vi "pelletpercents.vi"(6 "Run/Stop":bool, 8 "grading threshoulds":dbl[](array[numeric]), 11 "Sorted data":dbl[](array[numeric])) -> (2 "Percentage":dbl[](array[numeric]))   [LabVIEW 2019]
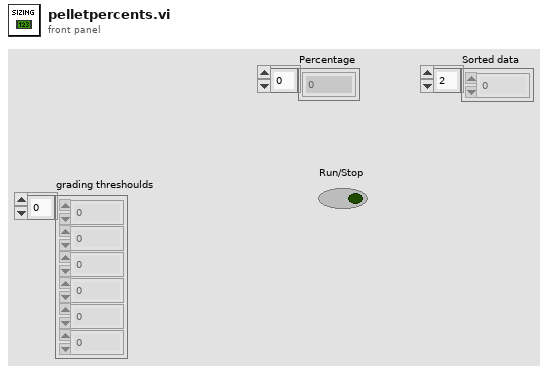
[diagram p1: front panel]
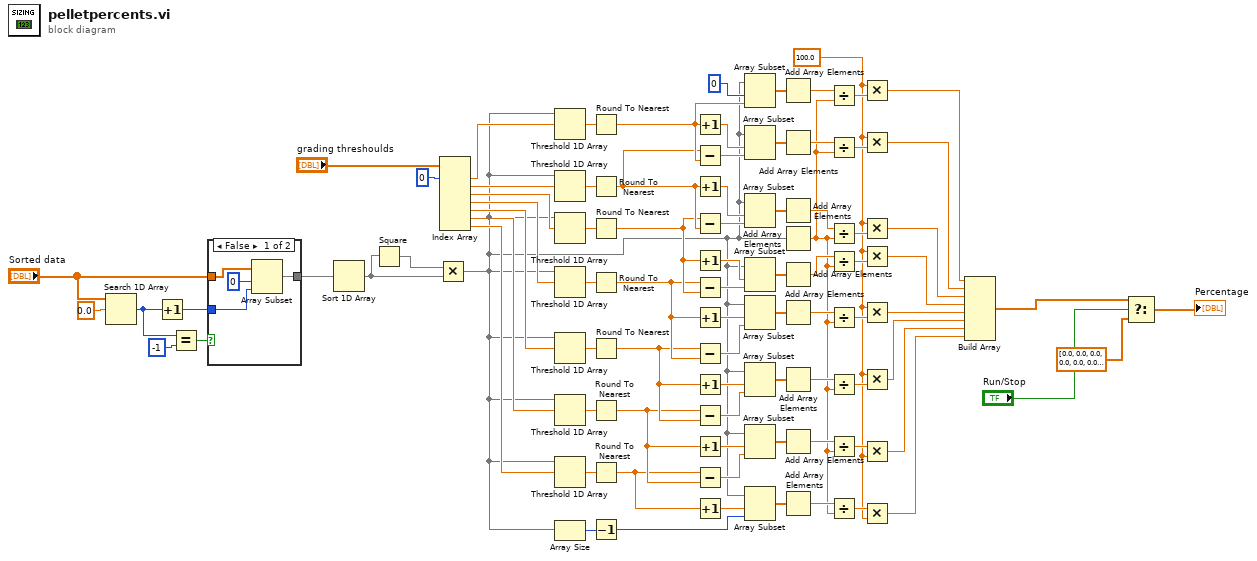
[diagram p0: block diagram]
diagram:
  w6 = 100.0 ("x")
  n1 = Search 1D Array(1D array="Sorted data", element=0.0) -> (index of element=w24:i32)  [unwired: 1 in]
  n2 = Increment(x=w24) -> (x+1=w23:i32)
  n3 = Equal?(x=w24, y=-1) -> (x = y?=w27:bool)
  n4 = case shown="False" w27 {
    tunnel: "Sorted data" -> [w91 w92]
    tunnel: [w88 w92] -> w25
    tunnel: w23 -> [w89 _]
    frame False {
      n5 = Array Subset(array=w91, index=0, length=w89) -> (w88:dbl[])
    }
    frame True {
    }
  }
  n6 = Sort 1D Array(array=w25) -> (sorted array=w30:dbl[])
  n7 = Square(x=w30) -> (x^2=w31:dbl[])
  n8 = Multiply(x=w31, y=w30) -> (x*y=w14:dbl[])
  n9 = Index Array(array="grading threshoulds", index #1=0 ("index")) -> (element #1=w22:dbl, element #2=w21:dbl, element #3=w20:dbl, element #4=w19:dbl, element #5=w18:dbl, element #6=w17:dbl, element #7=w15:dbl)  [unwired: 6 in]
  n10 = Threshold 1D Array(2:w22, 3:w14) -> (0:w79:dbl)  [unwired: 1 in]
  n11 = Threshold 1D Array(2:w21, 3:w14) -> (0:w86:dbl)  [unwired: 1 in]
  n12 = Threshold 1D Array(2:w20, 3:w14) -> (0:w85:dbl)  [unwired: 1 in]
  n13 = Threshold 1D Array(2:w19, 3:w14) -> (0:w84:dbl)  [unwired: 1 in]
  n14 = Threshold 1D Array(2:w18, 3:w14) -> (0:w83:dbl)  [unwired: 1 in]
  n15 = Threshold 1D Array(2:w17, 3:w14) -> (0:w82:dbl)  [unwired: 1 in]
  n16 = Threshold 1D Array(2:w15, 3:w14) -> (0:w16:dbl)  [unwired: 1 in]
  n17 = Array Size(array=w14) -> (size(s)=w55:i32)
  n18 = Round To Nearest(number=w79) -> (nearest integer value=w74:dbl)
  n19 = Round To Nearest(number=w86) -> (nearest integer value=w53:dbl)
  n20 = Round To Nearest(number=w85) -> (nearest integer value=w51:dbl)
  n21 = Round To Nearest(number=w84) -> (nearest integer value=w49:dbl)
  n22 = Round To Nearest(number=w83) -> (nearest integer value=w47:dbl)
  n23 = Round To Nearest(number=w82) -> (nearest integer value=w40:dbl)
  n24 = Round To Nearest(number=w16) -> (nearest integer value=w13:dbl)
  n25 = Decrement(x=w55) -> (x-1=w11:i32)
  n26 = Increment(x=w74) -> (x+1=w80:dbl)
  n27 = Subtract(x=w53, y=w74) -> (x-y=w54:dbl)
  n28 = Increment(x=w53) -> (x+1=w78:dbl)
  n29 = Subtract(x=w51, y=w53) -> (x-y=w52:dbl)
  n30 = Increment(x=w51) -> (x+1=w77:dbl)
  n31 = Subtract(x=w49, y=w51) -> (x-y=w50:dbl)
  n32 = Increment(x=w49) -> (x+1=w76:dbl)
  n33 = Subtract(x=w47, y=w49) -> (x-y=w48:dbl)
  n34 = Increment(x=w47) -> (x+1=w75:dbl)
  n35 = Subtract(x=w40, y=w47) -> (x-y=w46:dbl)
  n36 = Increment(x=w40) -> (x+1=w45:dbl)
  n37 = Subtract(x=w13, y=w40) -> (x-y=w44:dbl)
  n38 = Increment(x=w13) -> (x+1=w12:dbl)
  n39 = Array Subset(array=w14, index=0, length=w74) -> (w73:dbl[])
  n40 = Array Subset(array=w14, index=w80, length=w54) -> (w72:dbl[])
  n41 = Array Subset(array=w14, index=w78, length=w52) -> (w71:dbl[])
  n42 = Array Subset(array=w14, index=w77, length=w50) -> (w70:dbl[])
  n43 = Array Subset(array=w14, index=w76, length=w48) -> (w69:dbl[])
  n44 = Array Subset(array=w14, index=w75, length=w46) -> (w68:dbl[])
  n45 = Array Subset(array=w14, index=w45, length=w44) -> (w43:dbl[])
  n46 = Array Subset(array=w14, index=w12, length=w11) -> (w10:dbl[])
  n47 = Add Array Elements(numeric array=w73) -> (sum=w67:dbl)
  n48 = Add Array Elements(numeric array=w72) -> (sum=w66:dbl)
  n49 = Add Array Elements(numeric array=w71) -> (sum=w65:dbl)
  n50 = Add Array Elements(numeric array=w14) -> (sum=w8:dbl)
  n51 = Add Array Elements(numeric array=w70) -> (sum=w64:dbl)
  n52 = Add Array Elements(numeric array=w69) -> (sum=w63:dbl)
  n53 = Add Array Elements(numeric array=w68) -> (sum=w62:dbl)
  n54 = Add Array Elements(numeric array=w43) -> (sum=w42:dbl)
  n55 = Add Array Elements(numeric array=w10) -> (sum=w9:dbl)
  n56 = Divide(x=w67, y=w8) -> (x/y=w56:dbl)
  n57 = Divide(x=w66, y=w8) -> (x/y=w61:dbl)
  n58 = Divide(x=w65, y=w8) -> (x/y=w60:dbl)
  n59 = Divide(x=w64, y=w8) -> (x/y=w59:dbl)
  n60 = Divide(x=w63, y=w8) -> (x/y=w58:dbl)
  n61 = Divide(x=w62, y=w8) -> (x/y=w57:dbl)
  n62 = Divide(x=w42, y=w8) -> (x/y=w41:dbl)
  n63 = Divide(x=w9, y=w8) -> (x/y=w7:dbl)
  n64 = Multiply(x=w6, y=w56) -> (x*y=w39:dbl)
  n65 = Multiply(x=w6, y=w61) -> (x*y=w38:dbl)
  n66 = Multiply(x=w6, y=w60) -> (x*y=w37:dbl)
  n67 = Multiply(x=w6, y=w59) -> (x*y=w36:dbl)
  n68 = Multiply(x=w6, y=w58) -> (x*y=w35:dbl)
  n69 = Multiply(x=w6, y=w57) -> (x*y=w34:dbl)
  n70 = Multiply(x=w41, y=w6) -> (x*y=w33:dbl)
  n71 = Multiply(x=w7, y=w6) -> (x*y=w5:dbl)
  n72 = Build Array(w39, w38, w37, w36, w35, w34, w33, w5) -> (w1:dbl[])
  n73 = Select(t=w1, s="Run/Stop", f=dbl[] [0.0, 0.0, 0.0, 0.0, 0.0, 0.0, 0.0, 0.0] ("Percentage")) -> (s? t:f=→"Percentage":dbl[])
